vi "Simple Example.vi"() -> ()   [LabVIEW 2019]
uses:
  Test Bench Tools.lvlib
panel:
  out "Result":T1(array[cluster])
  in  "Stop":bool
  in  "Launch Test":bool
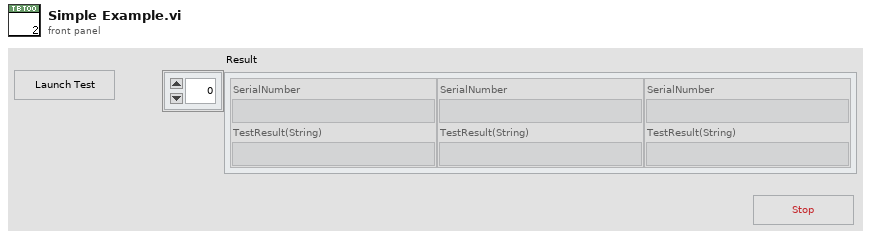
[diagram p1: front panel]
types:
  T1 = cluster{"SerialNumber":string, "TestResult(String)":string}[]
  T2 = enum16{"Station 1", "Station 2", "Station 3", "Station 4"}
  T3 = cluster{"new reference":refnum<k24>, "Array":refnum<k27>[], "Mgessage":refnum<user-event>}
  T4 = enum32{"Invalid", "Standard", "Closed", "Hidden", "Minimized", "Maximized"}
  T5 = enum32{"invalid app kind", "Development System", "Run Time System", "Student Edition", "Embedded LabVIEW", "Evaluation", "Custom"}
  T6 = cluster{"Core":cluster{"Current VI Reference":refnum<vi>, "Close Panel on Exit?":bool}, "Your Boolean data":bool, "Your string data":string, "hWnd":u32}
  T7 = cluster{"Current VI Reference":refnum<vi>, "Close Panel on Exit?":bool}
  T8 = enum16{"None", "Top", "Bottom", "Left", "Right", "Left-Top", "Left-Bottom", "Right-Top", "Right-Bottom"}[]
  T9 = cluster{"SerialNumber":string, "TestResult(String)":string}
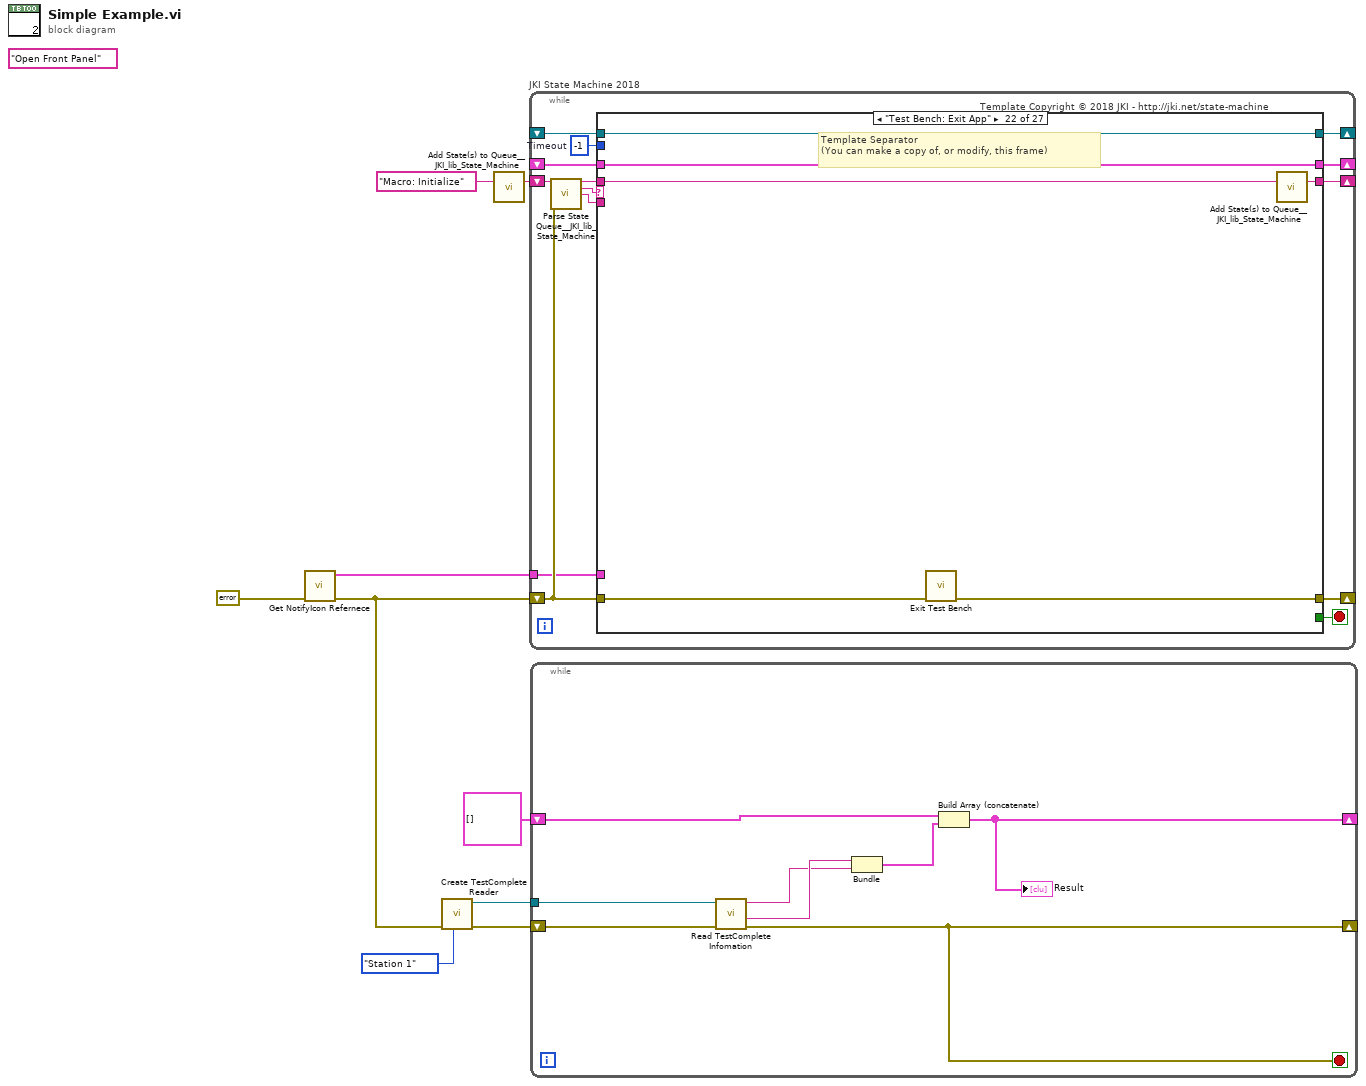
[diagram p0: block diagram]
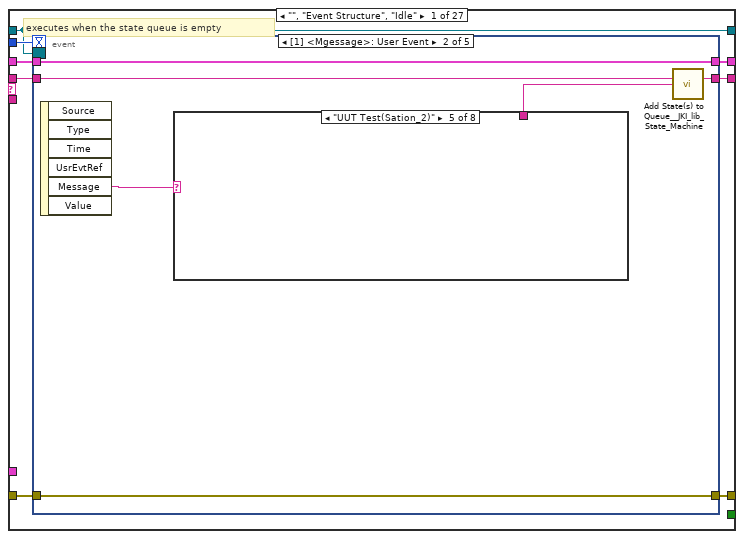
[diagram p2: hidden frame]
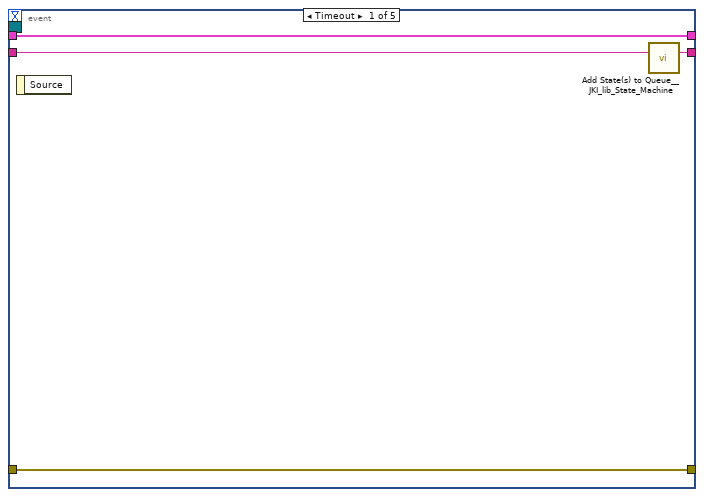
[diagram p3: hidden frame]
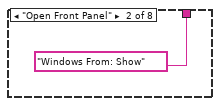
[diagram p5: hidden frame]
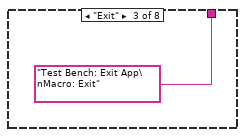
[diagram p6: hidden frame]
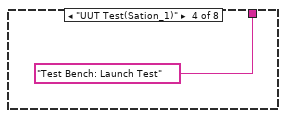
[diagram p7: hidden frame]
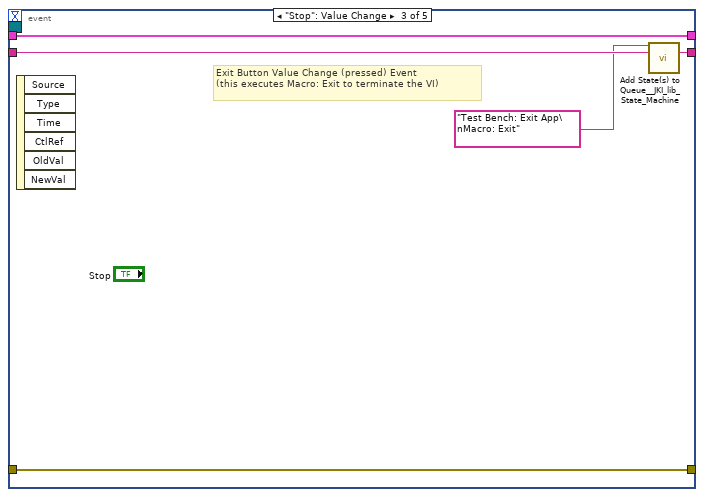
[diagram p11: hidden frame]
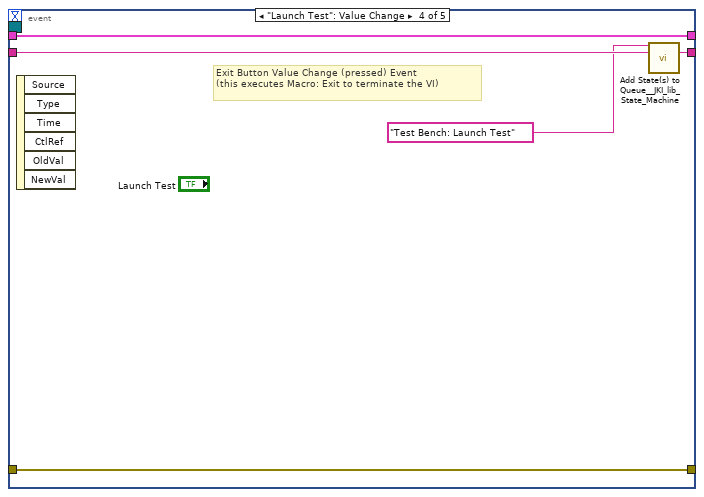
[diagram p12: hidden frame]
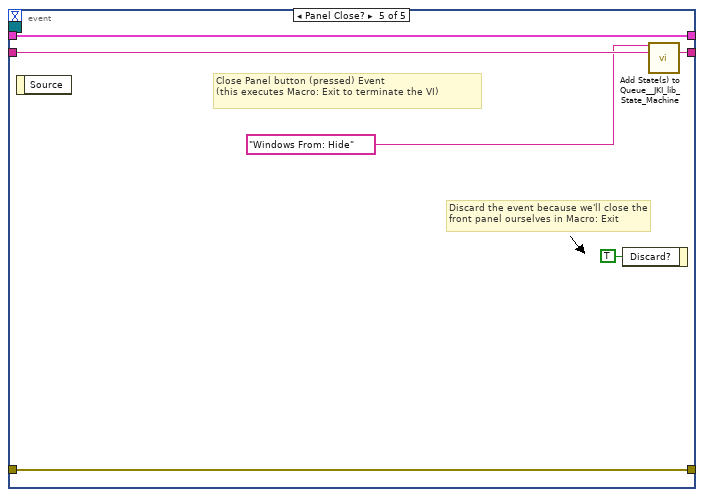
[diagram p13: hidden frame]
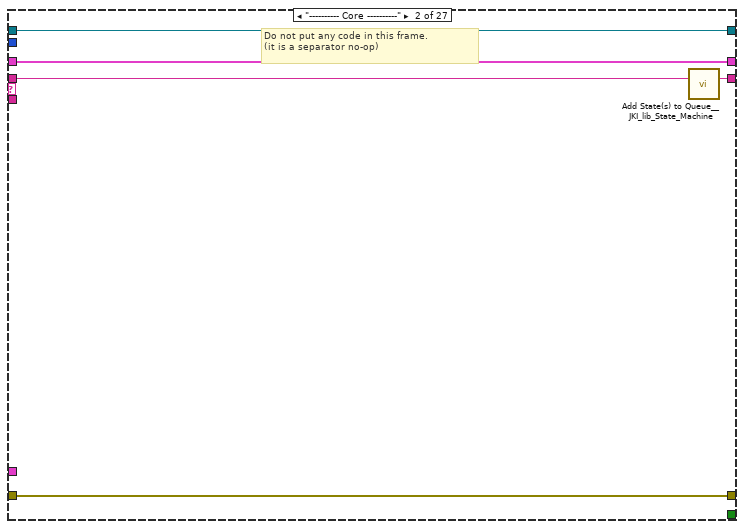
[diagram p14: hidden frame]
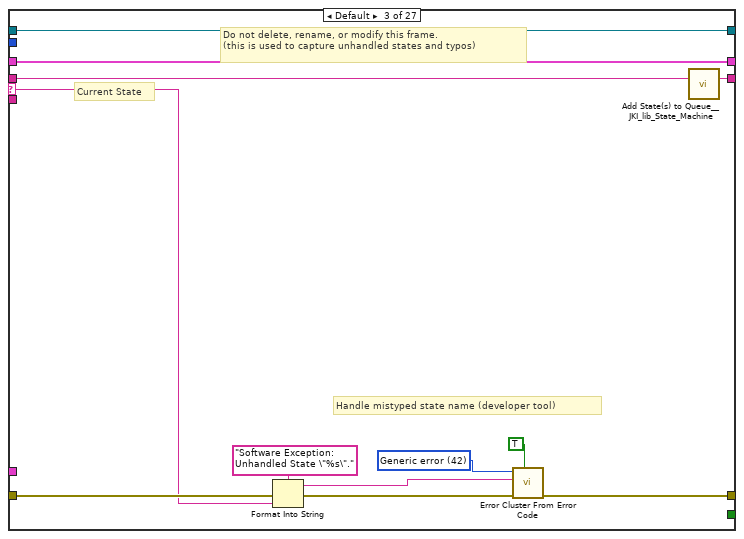
[diagram p15: hidden frame]
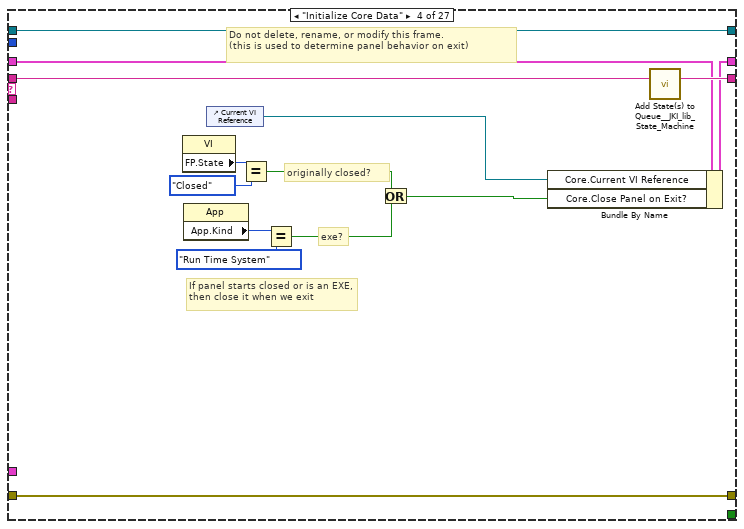
[diagram p16: hidden frame]
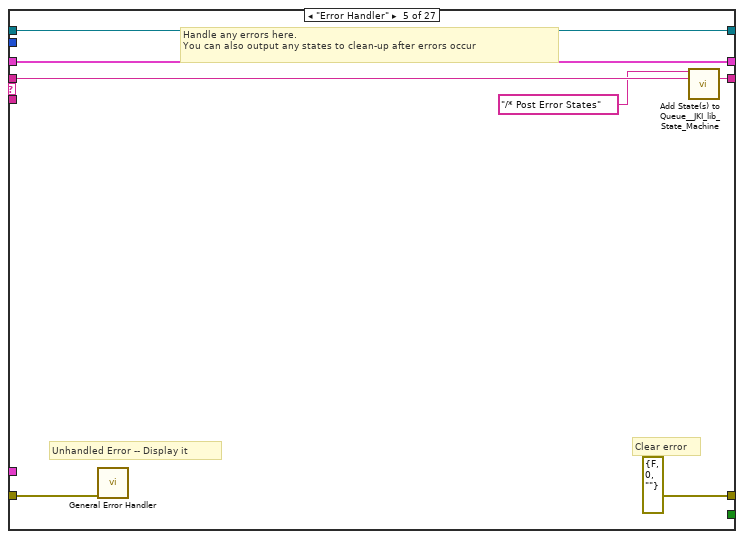
[diagram p17: hidden frame]
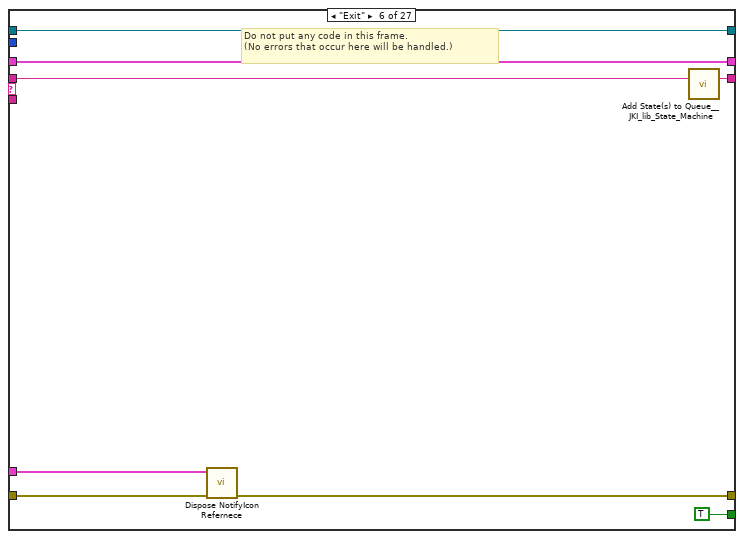
[diagram p18: hidden frame]
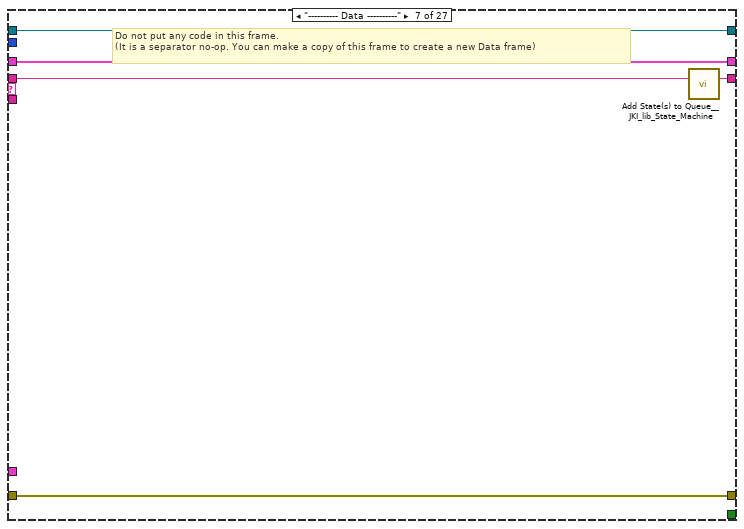
[diagram p19: hidden frame]
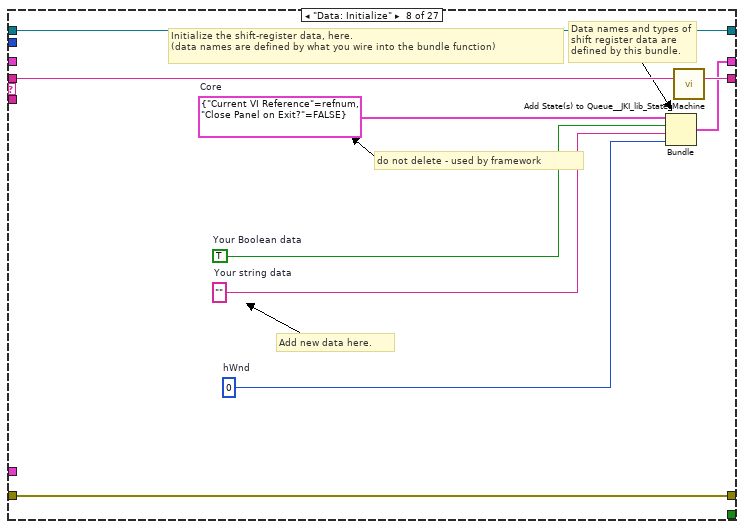
[diagram p20: hidden frame]
diagram:
  (unwired) "Open Front Panel" ("text")
  n1 = call "Get NotifyIcon Refernece.vi"("error in (no error)"=errorcluster {"status"=FALSE, "code"=0, "source"=""} ("error out")) -> ("error out"=w3:errorcluster, "reference out"=w2:T3)  [unwired: 9 in]
  n2 = call "Create TestComplete Reader.vi"("Station"=T2."Station 1", "error in (no error)"=w3) -> ("error out"=w7:errorcluster, "reader endpoint"=w5:refnum<k21>)  [unwired: 8 in]
  n3 = call <vilib>:"Add State(s) to Queue__JKI_lib_State_Machine.vi"("State(s) in (\"\")"="Macro: Initialize") -> ("States Out"=w9:string)  [unwired: 14 in]
  n4 = while "JKI State Machine 2018" {
    shift-right: [w16] -> _
    shift-left: _ -> [w15]
    shift-right: [w19] -> _
    shift-left: w3 -> [w13]
    shift-right: [w18] -> _
    shift-left: w9 -> [w20]
    shift-right: [w12] -> _
    shift-left: _ -> [w11]
    tunnel: w2 -> [w10]
    stop <- w17 stop-if-true
    w14 = -1  # Timeout
    # "Template Copyright © 2018 JKI - http://jki.net/state-machine"
    n5 = call <vilib>:"Parse State Queue__JKI_lib_State_Machine.vi"("State Queue"=w20, "Error In (no error)"=w13) -> ("Remaining States"=w22:string, "Current State"=w23:string, "Arguments"=w21:string)  [unwired: 11 in]
    n6 = case shown="\"Test Bench: Exit App\"" w23 {
      selector: w23 -> [_ _ w67 _ _ _ _ _ _ _ _ _ _ _ _ _ _ _ _ _ _ _ _ _ _ _ _]
      tunnel: w22 -> [w31 w65 w71 w91 w98 w106 w111 w120 w127 w132 w140 w146 w151 w156 w163 w175 w245 w251 w262 w267 w274 w280 w288 w293 w307 w324 w333]
      tunnel: w21 -> [_ _ _ _ _ _ _ _ _ _ _ _ _ _ w158 w169 _ _ _ _ _ _ _ _ _ _ _]
      tunnel: w15 -> [w29 w62 w69 w84 w95 w104 w108 _ w122 w129 w138 w144 w148 w154 w161 w171 w242 w248 w259 w264 w272 w278 w286 w290 w303 w321 w327]
      tunnel: [w28 w63 w73 w88 errorcluster {"status"=FALSE, "code"=0, "source"=""} ("error out") w99 w109 w117 w123 w130 w136 w141 w149 w153 w159 w172 w243 w249 w260 w265 w270 w276 w285 w289 w299 w309 w329] -> w19
      tunnel: w13 -> [w27 w63 w72 w88 w94 w100 w109 w117 w124 w130 w135 w142 w149 w153 w160 w173 w243 w249 w260 w265 w271 w277 w281 w289 w304 w315 w330]
      tunnel: [w30 w64 w70 w90 w97 w105 w110 w119 w126 w131 w139 w145 w150 w155 w162 w174 w244 w250 w261 w266 w273 w279 w287 w292 w306 w323 w332] -> w18
      tunnel: [_ _ _ _ _ TRUE _ _ _ _ _ _ _ _ _ _ _ _ _ _ _ _ _ _ _ _ _] -> w17
      tunnel: [w26 w62 w69 w89 w95 w104 w108 w118 w122 w129 w138 w144 w148 w154 w161 w171 w242 w248 w259 w264 w272 w278 w286 w290 w303 w321 w325] -> w16
      tunnel: w14 -> [w25 _ _ _ _ _ _ _ _ _ _ _ _ _ _ _ _ _ _ _ _ _ _ _ _ _ _]
      tunnel: [w24 w61 w66 w78 w92 w102 w107 w113 w121 w128 w137 w143 w147 w152 w157 w168 w241 w246 w252 w263 w269 w275 w283 w291 w305 w322 w331] -> w12
      tunnel: w11 -> [w24 w61 w66 w78 w92 w102 w107 w113 w121 w128 _ w143 w147 w152 w157 w168 w241 w246 w252 w263 w269 w275 w283 w291 w305 w322 w331]
      tunnel: w10 -> [_ _ _ _ _ w101 _ _ _ _ w134 _ _ _ _ _ _ _ _ _ _ _ _ _ _ _ _]
      frame "", "Event Structure", "Idle" {
        # "executes when the state queue is empty"
        n7 = event shown="[1] <Mgessage>: User Event" {
          selector: w24 -> [_ _ _ _ _]
          dyn-events: _ -> [_ _ _ _ _]
          timeout: w25 -> [_ _ _ _ _]
          tunnel: w31 -> [w35 w41 w49 w54 w60]
          tunnel: [w34 w40 w48 w53 w59] -> w30
          tunnel: w29 -> [w32 w38 w46 w51 w57]
          tunnel: [w33 w39 w47 w52 w58] -> w28
          tunnel: w27 -> [w33 w39 w47 w52 w58]
          tunnel: [w32 w38 w46 w51 w57] -> w26
          event Timeout {
            n8 = event-data() -> ()  [unwired: 1 in, 1 out]
            n9 = call <vilib>:"Add State(s) to Queue__JKI_lib_State_Machine.vi"("State(s) in (\"\")"=w35) -> ("States Out"=w34:string)  [unwired: 14 in]
          }
          event User Event {
            n10 = event-data() -> ("Message"=w37:string)  [unwired: 1 in, 5 out]
            n11 = case shown="\"UUT Test(Sation_2)\"" w37 {
              tunnel: [_ "Windows From: Show" "Test Bench: Exit App\nMacro: Exit" "Test Bench: Launch Test" _ _ _ _] -> w36
              frame "Idle", Default {
              }
              frame "Open Front Panel" {
              }
              frame "Exit" {
              }
              frame "UUT Test(Sation_1)" {
              }
              frame "UUT Test(Sation_2)" {
              }
              frame "UUT Test(Sation_3)" {
              }
              frame "UUT Test(Sation_4)" {
              }
              frame "Select Sequence(Sation_1)" {
              }
            }
            n12 = call <vilib>:"Add State(s) to Queue__JKI_lib_State_Machine.vi"("State(s) in (\"\")"=w41, "State(s) at Back (\"\")"=w36) -> ("States Out"=w40:string)  [unwired: 13 in]
          }
          event "Stop": Value Change {
            # "Exit Button Value Change (pressed) Event\n(this executes Macro: Exit to terminate the VI)"
            n13 = event-data() -> ()  [unwired: 1 in, 6 out]
            n14 = call <vilib>:"Add State(s) to Queue__JKI_lib_State_Machine.vi"("State(s) in Front (\"\")"="Test Bench: Exit App\nMacro: Exit", "State(s) in (\"\")"=w49) -> ("States Out"=w48:string)  [unwired: 13 in]
          }
          event "Launch Test": Value Change {
            # "Exit Button Value Change (pressed) Event\n(this executes Macro: Exit to terminate the VI)"
            n15 = event-data() -> ()  [unwired: 1 in, 6 out]
            n16 = call <vilib>:"Add State(s) to Queue__JKI_lib_State_Machine.vi"("State(s) in Front (\"\")"="Test Bench: Launch Test", "State(s) in (\"\")"=w54) -> ("States Out"=w53:string)  [unwired: 13 in]
          }
          event Panel Close? {
            # "Discard the event because we'll close the front panel ourselves in Macro: Exit"
            # "Close Panel button (pressed) Event\n(this executes Macro: Exit to terminate the VI)"
            n17 = event-data() -> ()  [unwired: 1 in, 1 out]
            n18 = event-data("Discard?"=TRUE) -> ()  [unwired: 1 in, 1 out]
            n19 = call <vilib>:"Add State(s) to Queue__JKI_lib_State_Machine.vi"("State(s) in Front (\"\")"="Windows From: Hide", "State(s) in (\"\")"=w60) -> ("States Out"=w59:string)  [unwired: 13 in]
          }
        }
      }
      frame "---------- Core ----------" {
        # "Do not put any code in this frame.\n(it is a separator no-op)"
        n20 = call <vilib>:"Add State(s) to Queue__JKI_lib_State_Machine.vi"("State(s) in (\"\")"=w65) -> ("States Out"=w64:string)  [unwired: 14 in]
      }
      frame Default {
        w76 = 42 items=["No error", "Argument error", "Memory is full", "Out of zone", "End of file", "File already open", "Generic file I/O error", "File not found", "File permission error", "Disk is full", "Duplicate path", "Too many files open", "System feature not enabled", "Resource file not found", "Cannot add resource", "Resource not found", "Image not found", "Image memory error", "Pen does not exist", "Config type invalid", "Config token not found", "Config parse error", "Config memory error", "Bad external code format", "Bad external code offset", "External code not present", "Null window", "Destroy window error", "Null menu", "Print aborted", "Bad print record", "Print driver error", "Windows error during printing", "Memory error during printing", "Print dialog error", "Generic print error", "Invalid device refnum", "Device not found", "Device parameter error", "Device unit error", "Cannot open device", "Device call aborted", "Generic error", "Cancelled by user", "Object ID too low", "Object ID too high", "Object not in heap", "Unknown heap", "Unknown object (invalid DefProc)", "Unknown object (DefProc not in table)", "Message out of range", "Invalid (null) method", "Unknown message", "Manager call not supported", "Bad address", "Network operation in progress", "Network operation timed out", "Connection is busy", "Network attribute not supported", "Network error", "Address in use", "System out of memory", "Connection aborted", "Connection refused", "Not connected", "Already connected", "Connection closed", "Initialization error (interapplication manager)", "Bad occurrence", "Wait on unbound occurrence handler", "Occurrence queue overflow", "Datalog type conflict", "Unused", "Unrecognized type (interapplication manager)", "Memory corrupt", "Failed to make temporary DLL", "Old CIN version", "Drag socket not found", "Failed to load drop-object", "Failed to register OLE object", "Failed to release OLE object", "Format specifier type mismatch", "Unknown format specifier", "Too few format specifiers", "Too many format specifiers", "Scan failed", "Newer CIN version", "Error converting to variant", "Runtime menu error", "Password tampered", "Variant attribute not found", "Incompatible variant data type", "Event data is not available", "Event Store is not present", "Occurrence is not found", "Event Queue is not created", "Event info is not available", "Refnum passed is NULL", "Error retrieving Class GUID", "Error retrieving CoClass GUID", "Error retrieving TypeLib GUID.", "Bad built application magic bytes.", "Specific driver is different from the specific driver associated with the Logical Name.", "There is no session opened to the class driver.", "Max Error", "MAX - Error with config objects", "MAX - Error loading configuration", "MAX - Group not supported"]
        # "Current State"
        # "Do not delete, rename, or modify this frame.\n(this is used to capture unhandled states and typos)"
        # "Handle mistyped state name (developer tool)"
        n21 = Format Into String(format string="Software Exception: Unhandled State \"%s\"." ("message"), error in=w72, w67) -> (resulting string=w75:string, error out=w74:errorcluster)  [unwired: 1 in]
        n22 = call <vilib>:"Error Cluster From Error Code.vi"("show call chain? (False)"=TRUE, "error in (no error)"=w74, "error message (\"\")"=w75, "error code (0)"=w76) -> ("error out"=w73:errorcluster)  [unwired: 5 in]
        n23 = call <vilib>:"Add State(s) to Queue__JKI_lib_State_Machine.vi"("State(s) in (\"\")"=w71) -> ("States Out"=w70:string)  [unwired: 14 in]
      }
      frame "Initialize Core Data" {
        # "Do not delete, rename, or modify this frame.\n(this is used to determine panel behavior on exit)"
        # "originally closed?"
        # "exe?"
        # "If panel starts closed or is an EXE, then close it when we exit"
        n24 = property class="VI"() -> ("FP.State"=w81:T4)  [unwired: 2 in, 2 out]
        n25 = property class="App"() -> ("App.Kind"=w87:T5)  [unwired: 2 in, 2 out]
        n26 = control-ref of="Current VI Reference"() -> (w82:refnum<vi>)
        n27 = Equal?(x=w81, y=T4."Closed" ("Front Panel Window:State")) -> (x = y?=w79:bool)
        n28 = Equal?(x=w87, y=T5."Run Time System" ("Application:Kind")) -> (x = y?=w85:bool)
        n29 = Or(x=w79, y=w85) -> (x .or. y?=w83:bool)
        n30 = Bundle By Name(cluster=w84, "Core.Current VI Reference"=w82, "Core.Close Panel on Exit?"=w83) -> (w89:T6)
        n31 = call <vilib>:"Add State(s) to Queue__JKI_lib_State_Machine.vi"("State(s) in (\"\")"=w91) -> ("States Out"=w90:string)  [unwired: 14 in]
      }
      frame "Error Handler" {
        # "Unhandled Error -- Display it"
        # "Handle any errors here.\nYou can also output any states to clean-up after errors occur"
        # "Clear error"
        n32 = call <vilib>:"General Error Handler.vi"("error in (no error)"=w94) -> ()  [unwired: 10 in, 5 out]
        n33 = call <vilib>:"Add State(s) to Queue__JKI_lib_State_Machine.vi"("State(s) in Front (\"\")"="/* Post Error States", "State(s) in (\"\")"=w98) -> ("States Out"=w97:string)  [unwired: 13 in]
      }
      frame "Exit" {
        # "Do not put any code in this frame.\n(No errors that occur here will be handled.)"
        n34 = call "Dispose NotifyIcon Refernece.vi"("error in (no error)"=w100, "reference"=w101) -> ("error out"=w99:errorcluster)  [unwired: 9 in]
        n35 = call <vilib>:"Add State(s) to Queue__JKI_lib_State_Machine.vi"("State(s) in (\"\")"=w106) -> ("States Out"=w105:string)  [unwired: 14 in]
      }
      frame "---------- Data ----------" {
        # "Do not put any code in this frame.\n(It is a separator no-op. You can make a copy of this frame to create a new Data frame)"
        n36 = call <vilib>:"Add State(s) to Queue__JKI_lib_State_Machine.vi"("State(s) in (\"\")"=w111) -> ("States Out"=w110:string)  [unwired: 14 in]
      }
      frame "Data: Initialize" {
        w112 = u32 0  # hWnd
        w114 = T7 {"Current VI Reference"=refnum, "Close Panel on Exit?"=FALSE}  # Core
        w116 = TRUE  # Your Boolean data
        w115 = ""  # Your string data
        # "do not delete - used by framework"
        # "Add new data here."
        # "Data names and types of shift register data are defined by this bundle."
        # "Initialize the shift-register data, here.\n(data names are defined by what you wire into the bundle function)"
        n37 = Bundle("Core"=w114, "Your Boolean data"=w116, "Your string data"=w115, "hWnd"=w112) -> (w118:T6)  [unwired: 1 in]
        n38 = call <vilib>:"Add State(s) to Queue__JKI_lib_State_Machine.vi"("State(s) in (\"\")"=w120) -> ("States Out"=w119:string)  [unwired: 14 in]
      }
      frame "Data: Cleanup" {
        # "Cleanup any data and references, here.\n(this is called automatically, by the Macro: Exit)"
        n39 = Unbundle By Name(w122) -> ("Core.Current VI Reference"=w125:refnum<vi>)
        n40 = Close Reference(reference=w125, error in (no error)=w124) -> (error out=w123:errorcluster)
        n41 = call <vilib>:"Add State(s) to Queue__JKI_lib_State_Machine.vi"("State(s) in (\"\")"=w127) -> ("States Out"=w126:string)  [unwired: 14 in]
      }
      frame "---------- Events ----------" {
        # "Do not put any code in this frame.\n(It is a separator no-op. You can make a copy of this frame to create a new UI frame)"
        n42 = call <vilib>:"Add State(s) to Queue__JKI_lib_State_Machine.vi"("State(s) in (\"\")"=w132) -> ("States Out"=w131:string)  [unwired: 14 in]
      }
      frame "Events: Register" {
        # "Do not put any code in this frame.\n(It is a separator no-op. You can make a copy of this frame to create a new UI frame)"
        n43 = Unbundle By Name(w134) -> ("Mgessage"=w133:refnum<user-event>)
        n44 = register-events(error in=w135, w133) -> (reference out=w137:refnum<event-registration>, error out=w136:errorcluster)  [unwired: 1 in]
        n45 = call <vilib>:"Add State(s) to Queue__JKI_lib_State_Machine.vi"("State(s) in (\"\")"=w140) -> ("States Out"=w139:string)  [unwired: 14 in]
      }
      frame "Events: Unregister" {
        # "Do not put any code in this frame.\n(It is a separator no-op. You can make a copy of this frame to create a new UI frame)"
        n46 = Unregister For Events(event registration refnum=w143, error in=w142) -> (error out=w141:errorcluster)
        n47 = call <vilib>:"Add State(s) to Queue__JKI_lib_State_Machine.vi"("State(s) in (\"\")"=w146) -> ("States Out"=w145:string)  [unwired: 14 in]
      }
      frame "---------- UI ----------" {
        # "Do not put any code in this frame.\n(It is a separator no-op. You can make a copy of this frame to create a new UI frame)"
        n48 = call <vilib>:"Add State(s) to Queue__JKI_lib_State_Machine.vi"("State(s) in (\"\")"=w151) -> ("States Out"=w150:string)  [unwired: 14 in]
      }
      frame "UI: Initialize" {
        # "Initialize the User Interface, here.\n(this is called automatically, by the Macro: Init)"
        n49 = call <vilib>:"Add State(s) to Queue__JKI_lib_State_Machine.vi"("State(s) in (\"\")"=w156) -> ("States Out"=w155:string)  [unwired: 14 in]
      }
      frame "UI: Cursor Set" {
        # "Argument"
        # "Set and Unset Cursor Busy.\n(Usage: \"UI: Cursor Set >> Busy|Idle\")"
        n50 = case shown="\"Idle\", Default" w158 {
          tunnel: w160 -> [w165 w167]
          tunnel: [w164 w166] -> w159
          frame "Idle", Default {
            n51 = call <vilib>:"Unset Busy.vi"("error in (no error)"=w165) -> ("error out"=w164:errorcluster)  [unwired: 10 in]
          }
          frame "Busy" {
            n52 = call <vilib>:"Set Busy.vi"("error in (no error)"=w167) -> ("error out"=w166:errorcluster)  [unwired: 9 in, 1 out]
          }
        }
        n53 = call <vilib>:"Add State(s) to Queue__JKI_lib_State_Machine.vi"("State(s) in (\"\")"=w163) -> ("States Out"=w162:string)  [unwired: 14 in]
      }
      frame "UI: Front Panel State" {
        # "Argument"
        # "Set Front Panel Open or Closed\n(Usage: \"UI: Front Panel State >> Open|Close\")"
        n54 = Unbundle By Name(w171) -> ("Core.Current VI Reference"=w170:refnum<vi>)
        n55 = case shown="\"Minimize\", \"Minimized\"" w169 {
          tunnel: w173 -> [w181 w196 w207 w220 w233]
          tunnel: [w183 w197 w209 w222 w235] -> w172
          tunnel: w170 -> [w182 w194 w208 w221 w234]
          frame "Open", "Standard", Default {
            w176 = T4."Standard" ("State")
            n56 = property class="VI"(reference=w182, error in=w181) -> (reference out=w179:refnum<vi>, error out=w180:errorcluster, "FP.State"=w178:T4)
            n57 = Not Equal?(x=w178, y=w176) -> (x != y?=w177:bool)
            n58 = case shown="True" w177 {
              tunnel: [w187 w189] -> w183
              tunnel: w180 -> [w186 w189]
              tunnel: w179 -> [w185 _]
              tunnel: w176 -> [w184 _]
              frame True {
                n59 = invoke class="VI" method="FP.Open"(reference=w185, error in=w186, "Activate"=TRUE, "State"=w184) -> (error out=w187:errorcluster)  [unwired: 1 in, 4 out]
              }
              frame False {
              }
            }
          }
          frame "Close", "Closed" {
            n60 = property class="VI"(reference=w194, error in=w196) -> (reference out=w193:refnum<vi>, error out=w195:errorcluster, "FP.State"=w191:T4)
            n61 = Not Equal?(x=w191, y=T4."Closed" ("Front Panel Window:State")) -> (x != y?=w190:bool)
            n62 = case shown="True" w190 {
              tunnel: [w198 w201] -> w197
              tunnel: w195 -> [w198 w200]
              tunnel: w193 -> [_ w199]
              frame False {
              }
              frame True {
                n63 = invoke class="VI" method="FP.Close"(reference=w199, error in=w200) -> (error out=w201:errorcluster)  [unwired: 1 in, 2 out]
              }
            }
          }
          frame "Hidden", "Hide" {
            w202 = T4."Hidden" ("State")
            n64 = property class="VI"(reference=w208, error in=w207) -> (reference out=w205:refnum<vi>, error out=w206:errorcluster, "FP.State"=w204:T4)
            n65 = Not Equal?(x=w204, y=w202) -> (x != y?=w203:bool)
            n66 = case shown="True" w203 {
              tunnel: [w213 w214] -> w209
              tunnel: w206 -> [w212 w214]
              tunnel: w205 -> [w211 _]
              tunnel: w202 -> [w210 _]
              frame True {
                n67 = invoke class="VI" method="FP.Open"(reference=w211, error in=w212, "State"=w210) -> (error out=w213:errorcluster)  [unwired: 2 in, 4 out]
              }
              frame False {
              }
            }
          }
          frame "Minimize", "Minimized" {
            w215 = T4."Minimized" ("State")
            n68 = property class="VI"(reference=w221, error in=w220) -> (reference out=w218:refnum<vi>, error out=w219:errorcluster, "FP.State"=w217:T4)
            n69 = Not Equal?(x=w217, y=w215) -> (x != y?=w216:bool)
            n70 = case shown="True" w216 {
              tunnel: [w226 w227] -> w222
              tunnel: w219 -> [w225 w227]
              tunnel: w218 -> [w224 _]
              tunnel: w215 -> [w223 _]
              frame True {
                n71 = invoke class="VI" method="FP.Open"(reference=w224, error in=w225, "State"=w223) -> (error out=w226:errorcluster)  [unwired: 2 in, 4 out]
              }
              frame False {
              }
            }
          }
          frame "Maximize", "Maximized" {
            w228 = T4."Maximized" ("State")
            n72 = property class="VI"(reference=w234, error in=w233) -> (reference out=w231:refnum<vi>, error out=w232:errorcluster, "FP.State"=w230:T4)
            n73 = Not Equal?(x=w230, y=w228) -> (x != y?=w229:bool)
            n74 = case shown="True" w229 {
              tunnel: [w239 w240] -> w235
              tunnel: w232 -> [w238 w240]
              tunnel: w231 -> [w237 _]
              tunnel: w228 -> [w236 _]
              frame True {
                n75 = invoke class="VI" method="FP.Open"(reference=w237, error in=w238, "State"=w236) -> (error out=w239:errorcluster)  [unwired: 2 in, 4 out]
              }
              frame False {
              }
            }
          }
        }
        n76 = call <vilib>:"Add State(s) to Queue__JKI_lib_State_Machine.vi"("State(s) in (\"\")"=w175) -> ("States Out"=w174:string)  [unwired: 14 in]
      }
      frame "---------- Macro ----------" {
        # "Do not put any code in this frame.\n(It is a separator no-op. You can make a copy of this frame to create a new Macro frame)"
        n77 = call <vilib>:"Add State(s) to Queue__JKI_lib_State_Machine.vi"("State(s) in (\"\")"=w245) -> ("States Out"=w244:string)  [unwired: 14 in]
      }
      frame "Macro: Initialize" {
        # "Initialization Macro\n(This is called once, when the VI starts)"
        n78 = call <vilib>:"Add State(s) to Queue__JKI_lib_State_Machine.vi"("State(s) in Front (\"\")"="Data: Initialize\nInitialize Core Data\nEvents: Register\nUI: Initialize\nUI: Front Panel State >> Open\nTest Bench: Launch Test Bench\nWindows From: Find Windows\nWindows From: Hide", "State(s) in (\"\")"=w251) -> ("States Out"=w250:string)  [unwired: 13 in]
      }
      frame "Macro: Exit" {
        # "Exit Macro\n(This is called once, when the VI exits)"
        n79 = Unbundle By Name(w259) -> ("Core.Close Panel on Exit?"=w258:bool)
        n80 = Select(t="UI: Front Panel State >> Close", s=w258, f="") -> (s? t:f=w255:string)
        n81 = call <vilib>:"Add State(s) to Queue__JKI_lib_State_Machine.vi"("State(s) in (\"\")"=w255, "State(s) at Back (\"\")"="Data: Cleanup\nEvents: Unregister\nExit") -> ("States Out"=w253:string)  [unwired: 13 in]
        n82 = call <vilib>:"Add State(s) to Queue__JKI_lib_State_Machine.vi"("State(s) in Front (\"\")"=w253, "State(s) in (\"\")"=w262) -> ("States Out"=w261:string)  [unwired: 13 in]
      }
      frame "---------- Test Bench ----------" {
        # "Template Separator\n(You can make a copy of, or modify, this frame)"
        n83 = call <vilib>:"Add State(s) to Queue__JKI_lib_State_Machine.vi"("State(s) in (\"\")"=w267) -> ("States Out"=w266:string)  [unwired: 14 in]
      }
      frame "Test Bench: Launch Test Bench" {
        w268 = T8 [enum."None"] items=["None", "Top", "Bottom", "Left", "Right", "Left-Top", "Left-Bottom", "Right-Top", "Right-Bottom"] ("Position")
        # "Template Separator\n(You can make a copy of, or modify, this frame)"
        n84 = call "Launch Test Bench.vi"("Position"=w268, "error in (no error)"=w271) -> ("error out"=w270:errorcluster)  [unwired: 9 in]
        n85 = call <vilib>:"Add State(s) to Queue__JKI_lib_State_Machine.vi"("State(s) in (\"\")"=w274) -> ("States Out"=w273:string)  [unwired: 14 in]
      }
      frame "Test Bench: Exit App" {
        # "Template Separator\n(You can make a copy of, or modify, this frame)"
        n86 = call "Exit Test Bench.vi"("error in (no error)"=w277) -> ("error out"=w276:errorcluster)  [unwired: 10 in]
        n87 = call <vilib>:"Add State(s) to Queue__JKI_lib_State_Machine.vi"("State(s) in (\"\")"=w280) -> ("States Out"=w279:string)  [unwired: 14 in]
      }
      frame "Test Bench: Launch Test" {
        # "Template Separator\n(You can make a copy of, or modify, this frame)"
        n88 = property on="Result" class="Arr (strict)"("Value"=T1 [] ("Array")) -> ()  [unwired: 2 in, 2 out]
        n89 = call "Launch Test.vi"("Station"=T2."Station 1", "error in (no error)"=w281) -> ("error out"=w285:errorcluster)  [unwired: 9 in]
        n90 = call <vilib>:"Add State(s) to Queue__JKI_lib_State_Machine.vi"("State(s) in (\"\")"=w288) -> ("States Out"=w287:string)  [unwired: 14 in]
      }
      frame "---------- Windows From ----------" {
        # "Template Separator\n(You can make a copy of, or modify, this frame)"
        n91 = call <vilib>:"Add State(s) to Queue__JKI_lib_State_Machine.vi"("State(s) in (\"\")"=w293) -> ("States Out"=w292:string)  [unwired: 14 in]
      }
      frame "Windows From: Show" {
        w295 = u32 2 items=["SWP_ASYNCWINDOWPOS"=16384, "SWP_DEFERERASE"=8192, "SWP_DRAWFRAME"=32, "SWP_HIDEWINDOW"=128, "SWP_NOACTIVATE"=16, "SWP_NOCOPYBITS"=256, "SWP_NOMOVE"=2, "SWP_NOOWNERZORDER"=512, "SWP_NOREDRAW"=8, "SWP_NOSENDCHANGING"=1024, "SWP_NOSIZE"=1, "SWP_NOZORDER"=4, "SWP_SHOWWINDOW"=64] ("uFlags")
        w296 = u32 1 items=["SWP_ASYNCWINDOWPOS"=16384, "SWP_DEFERERASE"=8192, "SWP_DRAWFRAME"=32, "SWP_HIDEWINDOW"=128, "SWP_NOACTIVATE"=16, "SWP_NOCOPYBITS"=256, "SWP_NOMOVE"=2, "SWP_NOOWNERZORDER"=512, "SWP_NOREDRAW"=8, "SWP_NOSENDCHANGING"=1024, "SWP_NOSIZE"=1, "SWP_NOZORDER"=4, "SWP_SHOWWINDOW"=64] ("uFlags")
        # "Template Separator\n(You can make a copy of, or modify, this frame)"
        n92 = Unbundle By Name(w303) -> ("hWnd"=w302:u32)
        n93 = Or(x=w296, y=w295) -> (x .or. y?=w294:u32)
        n94 = call "Show Windows.vi"("nCmdShow"="SW_SHOWNORMAL", "error in (no error)"=w304, "hWnd"=w302) -> ("error out"=w300:errorcluster, "hWnd out"=w298:u32)  [unwired: 7 in]
        n95 = call "Set Windows Position.vi"("error in (no error)"=w300, "uFlags"=w294, "hWndInsertAfter"="-1", "hWnd"=w298) -> ("error out"=w299:errorcluster)  [unwired: 6 in, 1 out]
        n96 = call <vilib>:"Add State(s) to Queue__JKI_lib_State_Machine.vi"("State(s) in (\"\")"=w307) -> ("States Out"=w306:string)  [unwired: 14 in]
      }
      frame "Windows From: Hide" {
        w318 = u32 2 items=["SWP_ASYNCWINDOWPOS"=16384, "SWP_DEFERERASE"=8192, "SWP_DRAWFRAME"=32, "SWP_HIDEWINDOW"=128, "SWP_NOACTIVATE"=16, "SWP_NOCOPYBITS"=256, "SWP_NOMOVE"=2, "SWP_NOOWNERZORDER"=512, "SWP_NOREDRAW"=8, "SWP_NOSENDCHANGING"=1024, "SWP_NOSIZE"=1, "SWP_NOZORDER"=4, "SWP_SHOWWINDOW"=64] ("uFlags")
        w319 = u32 1 items=["SWP_ASYNCWINDOWPOS"=16384, "SWP_DEFERERASE"=8192, "SWP_DRAWFRAME"=32, "SWP_HIDEWINDOW"=128, "SWP_NOACTIVATE"=16, "SWP_NOCOPYBITS"=256, "SWP_NOMOVE"=2, "SWP_NOOWNERZORDER"=512, "SWP_NOREDRAW"=8, "SWP_NOSENDCHANGING"=1024, "SWP_NOSIZE"=1, "SWP_NOZORDER"=4, "SWP_SHOWWINDOW"=64] ("uFlags")
        # "Template Separator\n(You can make a copy of, or modify, this frame)"
        n97 = Unbundle By Name(w321) -> ("hWnd"=w316:u32)
        n98 = Or(x=w319, y=w318) -> (x .or. y?=w317:u32)
        n99 = call "Set Windows Position.vi"("error in (no error)"=w315, "uFlags"=w317, "hWndInsertAfter"="-2", "hWnd"=w316) -> ("error out"=w313:errorcluster, "hWnd out"=w314:u32)  [unwired: 6 in]
        n100 = call "Show Windows.vi"("nCmdShow"="SW_SHOWMINIMIZED", "error in (no error)"=w313, "hWnd"=w314) -> ("error out"=w311:errorcluster, "hWnd out"=w310:u32)  [unwired: 7 in]
        n101 = call "Show Windows.vi"("nCmdShow"="SW_HIDE", "error in (no error)"=w311, "hWnd"=w310) -> ("error out"=w309:errorcluster)  [unwired: 7 in, 1 out]
        n102 = call <vilib>:"Add State(s) to Queue__JKI_lib_State_Machine.vi"("State(s) in (\"\")"=w324) -> ("States Out"=w323:string)  [unwired: 14 in]
      }
      frame "Windows From: Find Windows" {
        # "Template Separator\n(You can make a copy of, or modify, this frame)"
        n103 = Unbundle By Name(w327) -> ("Core.Current VI Reference"=w328:refnum<vi>)
        n104 = call "Find Windows.vi"("error in (no error)"=w330, "VI reference"=w328) -> ("error out"=w329:errorcluster, "hWnd"=w326:u32)  [unwired: 8 in]
        n105 = Bundle By Name(cluster=w327, "hWnd"=w326) -> (w325:T6)
        n106 = call <vilib>:"Add State(s) to Queue__JKI_lib_State_Machine.vi"("State(s) in (\"\")"=w333) -> ("States Out"=w332:string)  [unwired: 14 in]
      }
    }
  }
  n107 = while {
    tunnel: w5 -> [w341]
    shift-right: [w339] -> _
    shift-left: w7 -> [w340]
    shift-right: [w334] -> _
    shift-left: T1 [] -> [w335]
    stop <- w339 stop-if-true
    n108 = call "Read TestComplete Infomation.vi"("error in (no error)"=w340, "endpoint in"=w341) -> ("error out"=w339:errorcluster, "SerialNumber"=w338:string, "TestResult(String)"=w337:string)  [unwired: 5 in, 2 out]
    n109 = Bundle("SerialNumber"=w338, "TestResult(String)"=w337) -> (w336:T9)  [unwired: 1 in]
    n110 = Build Array (concatenate)(w335, w336) -> (w334:T1)
    "Result" <- w334
  }
